vi "PH_BackreflectionMeas.calc Status.vi"(0 "i ref in":refnum<vi>, 5 "error in":errorcluster) -> (14 "i ref out":refnum<vi>, 19 "error out":errorcluster)   [LabVIEW 2014, in "PH_BackreflectionMeas.lvlib"]
uses:
  PH_BackreflectionMeas.lvlib
  PH_Basics/PH_StatusHandler/PH_StatusHandler.Status.ctl
  PH_Devices/PH_TKTDS-30xx/PH_TKTDS-30xx.lvlib
  PH_Basics/PH_Common/PH_Common.lvlib
  PH_Basics/PH_StatusHandler/PH_StatusHandler.lvlib
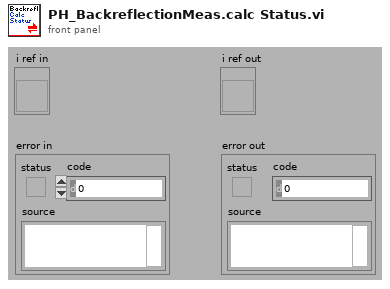
[diagram p1: front panel]
types:
  T1 = typedef "PH_BackreflectionMeas.lvlib/PH_BackreflectionMeas.i attribute.ctl" = cluster{"GUI Refs":cluster{"Get Data":refnum<vi>, "BR State":refnum<vi>, "Reset warning":refnum<vi>, "Low Energy Graph":refnum<vi>}, "Status":cluster{"Reset Warning":bool}, "Default Low Energy Chan Settings":T2, "Default High Energy Chan Settings":T2, "Default Trigger Settings":T3, "Default Acqu Settings":T4, "Limit [V]":dbl}
  T2 = typedef "PH_TKTDS-30xx.lvlib/PH_TKTDS-30xx.Channel Config.ctl" = cluster{"Channel Name":string, "Input Impedance":string, "Max Input Frequency":string, "Vertical Coupling":i32, "Channel Enabled":bool, "Probe Attenuation":dbl, "Vertical Range":dbl, "Vertical Offset":dbl}
  T3 = typedef "PH_TKTDS-30xx.lvlib/PH_TKTDS-30xx.Trigger Config.ctl" = cluster{"Source":string, "Slope":i32, "Level [V]":dbl}
  T4 = typedef "PH_TKTDS-30xx.lvlib/PH_TKTDS-30xx.Acquisition Config.ctl" = cluster{"Time base":dbl, "Record Length":u16, "Start Time":dbl, "Type":i32, "Continuous":bool}
  T5 = typedef "PH_TKTDS-30xx.lvlib/PH_TKTDS-30xx.i attribute.ctl" = cluster{"Default VISA Resource":string, "VISA Resource Name":refnum<visa-resource-name>, "Revision":cluster{"Instrument Driver":string, "Instrument Firmware":string}, "Selftest":cluster{"Result":u32, "Message":string}, "Channels":T2[], "Trigger Configuration":T3, "Acquisition Configuration":T4, "Fetched Waveforms":T6[], "GUI Refs":T7, "GUI Refs Channels":refnum<vi>[], "State":T8, "Error Message":string, "Allow Prdc Loop?":bool}
  T6 = typedef "PH_TKTDS-30xx.lvlib/PH_TKTDS-30xx.fetched Waveform.ctl" = cluster{"Source":string, "Actual Points":u32, "Initial X":dbl, "X Increment":dbl, "Waveform Array":dbl[]}
  T7 = typedef "PH_TKTDS-30xx.lvlib/PH_TKTDS-30xx.GUI Refs.ctl" = cluster{"Trigger":refnum<vi>, "Acquisition":refnum<vi>, "Graph":refnum<vi>, "State":refnum<vi>, "Delete":refnum<vi>, "Channel to be positioned":refnum<vi>, "Postion":refnum<vi>, "Display Intensity":refnum<vi>, "VISA Resource":refnum<vi>}
  T8 = typedef "PH_StatusHandler.lvlib/PH_StatusHandler.Status.ctl" = i16
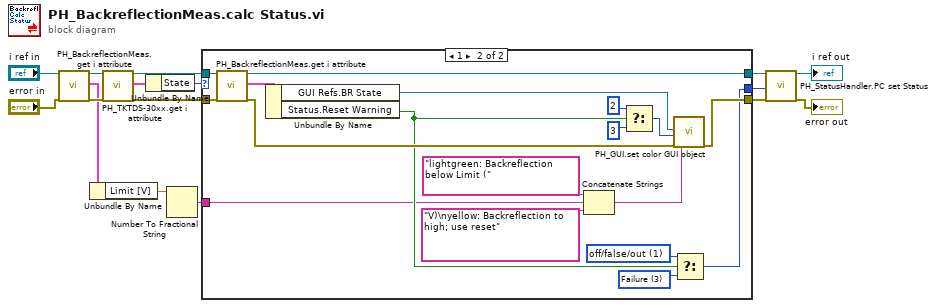
[diagram p0: block diagram]
diagram:
  n1 = call "PH_BackreflectionMeas.get i attribute.vi"("i ref in"="i ref in", "error in (no error)"="error in") -> ("i ref out"=w6:refnum<vi>, "i attribute"=w1:T1, "error out"=w5:errorcluster)  [unwired: 15 in]
  n2 = Unbundle By Name(w1) -> ("Limit [V]"=w2:dbl)
  n3 = call "PH_TKTDS-30xx.get i attribute.vi"("i ref in"=w6, "error in (no error)"=w5) -> ("i ref out"=w12:refnum<vi>, "i attribute"=w13:T5, "error out"=w9:errorcluster)  [unwired: 15 in]
  n4 = Unbundle By Name(w13) -> ("State"=w8:T8)
  n5 = Number To Fractional String(number=w2) -> (F-format string=w3:string)  [unwired: 3 in]
  n6 = case shown="1" w8 {
    selector: w8 -> [w19 _]
    tunnel: w12 -> [w18 w37]
    tunnel: [w17 w36] -> w11
    tunnel: [w18 w32] -> w10
    tunnel: w9 -> [w17 w31]
    tunnel: [w19 w24] -> w7
    tunnel: w3 -> [_ w22]
    frame Default {
    }
    frame 1 {
      w26 = T8 3 items=["no info", "off/false/out", "on/true/in", "Failure", "Alarm", "Status 1", "Status 2", "Status 3"] ("f")
      w27 = T8 1 items=["no info", "off/false/out", "on/true/in", "Failure", "Alarm", "Status 1", "Status 2", "Status 3"] ("State")
      n7 = call "PH_BackreflectionMeas.get i attribute.vi"("i ref in"=w37, "error in (no error)"=w31) -> ("i ref out"=w32:refnum<vi>, "i attribute"=w29:T1, "error out"=w30:errorcluster)  [unwired: 15 in]
      n8 = Unbundle By Name(w29) -> ("GUI Refs.BR State"=w28:refnum<vi>, "Status.Reset Warning"=w25:bool)
      n9 = Concatenate Strings("lightgreen: Backreflection below Limit (" ("Tip Strip (N/A)"), w22, "V)\nyellow: Backreflection to high; use reset" ("Tip Strip (N/A)")) -> (w23:string)
      n10 = Select(t=2 ("State"), s=w25, f=3) -> (s? t:f=w33:i32)
      n11 = call "PH_GUI.set color GUI object.vi"("GUI object Ref"=w28, "State"=w33, "error in (no error)"=w30, "Tip Strip (N/A)"=w23) -> ("error out"=w36:errorcluster)  [unwired: 15 in]
      n12 = Select(t=w27, s=w25, f=w26) -> (s? t:f=w24:T8)
    }
  }
  n13 = call "PH_StatusHandler.PC set Status.vi"("i ref in"=w10, "Status"=w7, "error in (no error)"=w11) -> ("i ref out"=→"i ref out":refnum<vi>, "error out"=→"error out":errorcluster)  [unwired: 15 in]
